vi "globalSetUp.vi"(8 "error in":errorcluster, 11 "Logging Loopback":refnum<class "Logging Loopback.lvclass">) -> (0 "error out":errorcluster, 3 "Logging Loopback out":refnum<class "Logging Loopback.lvclass">)   [LabVIEW 2020, in "Logging Loopback.lvclass"]
doc: "setUp runs prior to the test method during test execution. Use this method to initialize any object data required by your tests."
uses:
  Logging Loopback.lvclass
  Loopback/Loopback.lvclass
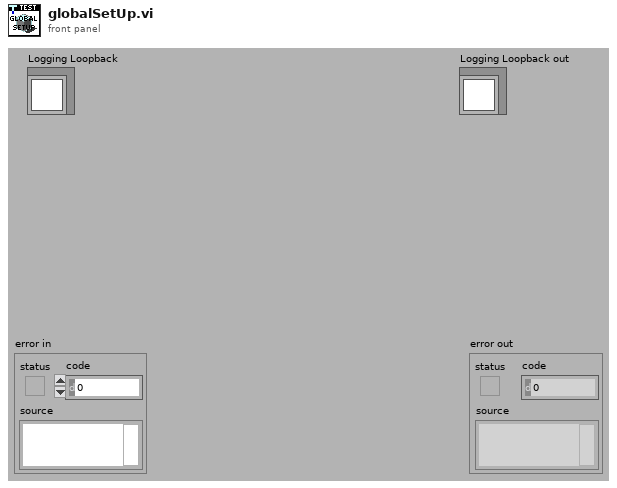
[diagram p1: front panel]
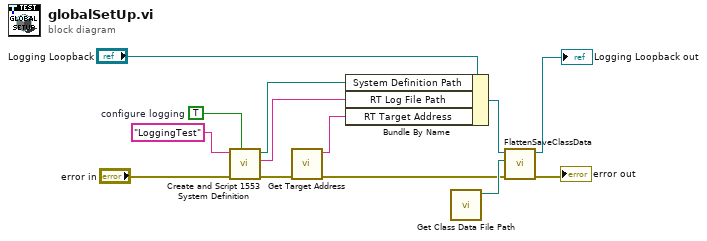
[diagram p0: block diagram]
diagram:
  w6 = TRUE  # configure logging
  n1 = call "Create and Script 1553 System Definition.vi"("configure logging"=w6, "error in"="error in", "System Definition Name"="LoggingTest") -> ("error out"=w4:errorcluster, "log file path"=w3:string, "System Definition Path"=w12:path)  [unwired: 6 in]
  n2 = call "Get Target Address.vi"("error in (no error)"=w4) -> ("error out"=w2:errorcluster, "target address"=w1:string)  [unwired: 9 in]
  n3 = Bundle By Name(cluster="Logging Loopback", "System Definition Path"=w12, "RT Log File Path"=w3, "RT Target Address"=w1) -> (w11:refnum<class "Logging Loopback.lvclass">)
  n4 = call "Get Class Data File Path.vi"() -> ("Class Data File Path"=w13:path)  [unwired: 11 in]
  n5 = call-dynamic "FlattenSaveClassData.vi"("error in"=w2, "Class Data File Path"=w13, "VeriStandTestCase in"=w11) -> ("error out"=→"error out":errorcluster, "VeriStandTestCase out"=→"Logging Loopback out":refnum<class "Logging Loopback.lvclass">)  [unwired: 7 in]
